vi "Variabila_Globala.vi"() -> ()   [LabVIEW 2024]
panel:
  out "Datele citite":string[](array[string])
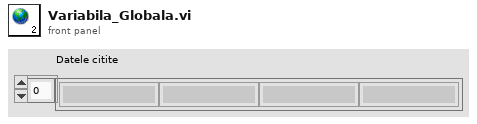
[diagram p1: front panel]
diagram:
